vi "Details Display Dialog.vi"(0 "Source":string caption="源", 1 "Start":i32[](array[numeric]) caption="开始", 2 "Length":i32[](array[numeric]) caption="长度", 3 "code":i32 caption="代码", 4 "Show Link":bool caption="显示链接", 5 "Details":string="问题原因" caption="详细信息", 7 "dialog type":T3 caption="对话框类型", 9 "Error or Warning":bool caption="错误或警告", 11 "contname":string="继续" caption="控件名", 12 "stopname":string="停止" caption="停止名", 13 "okname":string="确定" caption="确定名", 14 "Tag Found?":T1 caption="找到标识符？") -> (15 "stop event propagated":bool caption="停止被传递的事件")   [LabVIEW 2018]
uses:
  DialogTypeEnum.ctl
  ErrWarn.ctl
  TagReturnType.ctl
  eventvkey.ctl
panel:
  in  "Search ni.com":bool caption="搜索ni.com"
  in  "truncated message":string="（已删节的源）" caption="删节后消息"
  in  "truncated & CH message":string="（已删节的源；见即时帮助窗口）" caption="删节与CH消息"
  out "Source of Error":string caption="错误来源"
  out "scrollbar text":string caption="滚动条文本"
  in  "Test for size":string caption="大小测试"
  out "text":string caption="文本"
  out "Error or Warning Glyph":T2=TRUE caption="错误或警告图形标记"
  in  "OK":bool caption="确定"
  in  "Stop":bool caption="停止"
  in  "Continue":bool caption="继续"
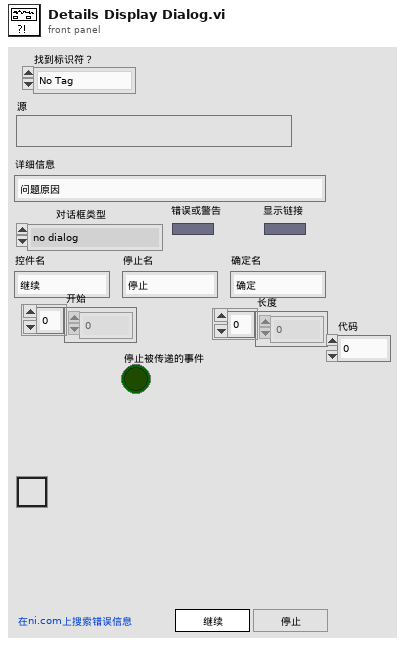
[diagram p1: front panel]
types:
  T1 = typedef "TagReturnType.ctl" = enum16{"No Tag", "<err>", "<append>"}
  T2 = typedef "ErrWarn.ctl" = bool
  T3 = typedef "DialogTypeEnum.ctl" = enum16{"no dialog", "OK message", "continue or stop message", "auto error handling dialog", "OK message + warnings", "continue/stop + warnings"}
  T4 = typedef "eventvkey.ctl" = enum16{"ASCII", "Enter", "Return", "Shift", "Ctrl", "Alt", "Cmd", "Opt", "Caps", "NumLock", "Clear", "Break", "Up", "Down", "Left", "Right", "Insert", "Delete", "Home", "End", "PageUp", "PageDown", "Escape", "Help", "Pause", "ScrollLock", "F1", "F2", "F3", "F4", "F5", "F6", "F7", "F8", "F9", "F10", "F11", "F12", "F13", "F14", "F15", "F16", "F17", "F18", "F19", "F20", "F21", "F22", "F23", "F24", "Play", "VolumeUp", "VolumeDown", "Mute", "Two Byte Char"}
  T5 = typedef "LVRectTypeDef.ctl" = cluster{"Left":i16, "Top":i16, "Right":i16, "Bottom":i16}
  T6 = cluster{"Control":bool, "Shift":bool, "Key":string}
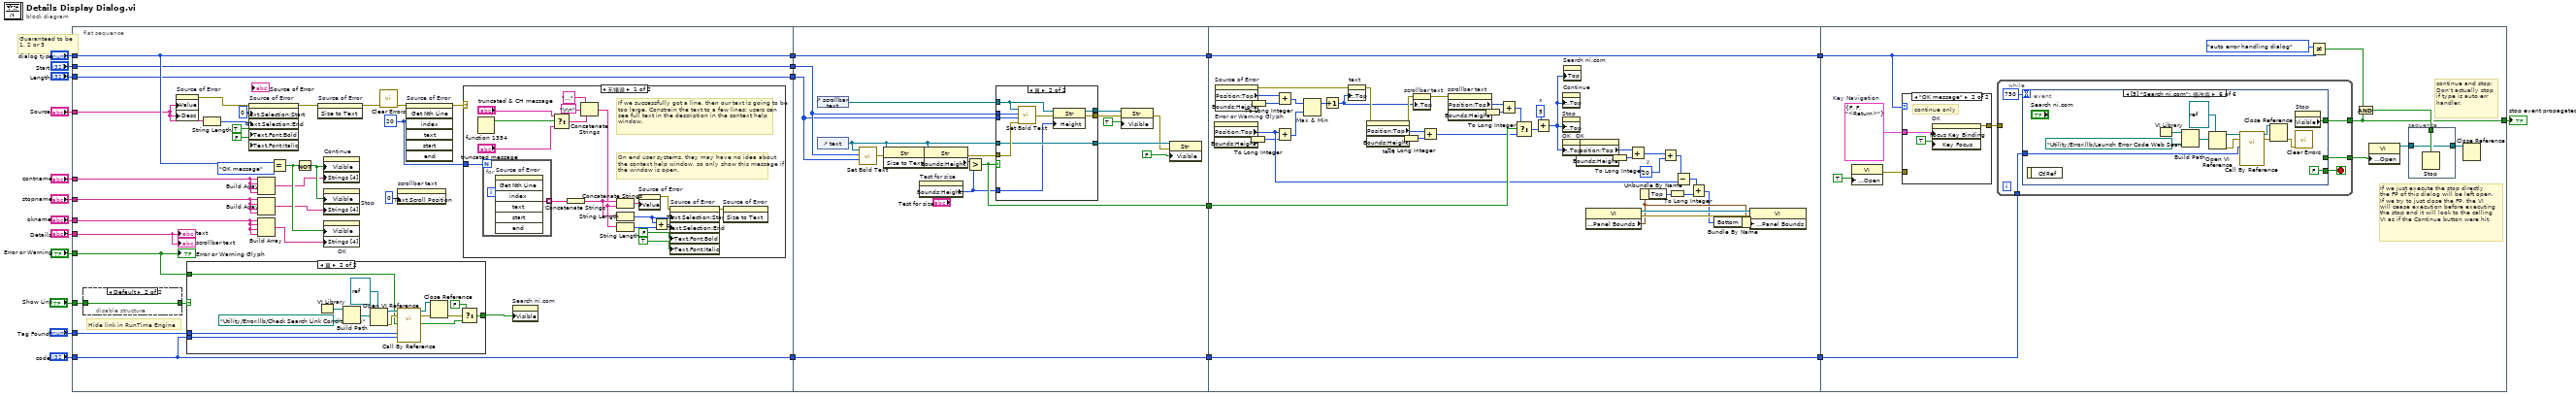
[diagram p0: block diagram]
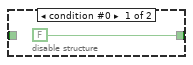
[diagram p2: hidden frame]
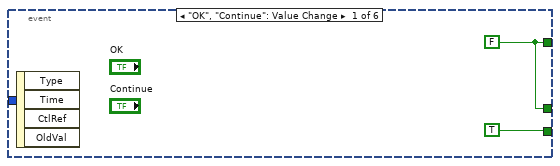
[diagram p6: hidden frame]
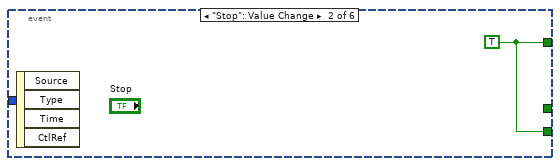
[diagram p7: hidden frame]
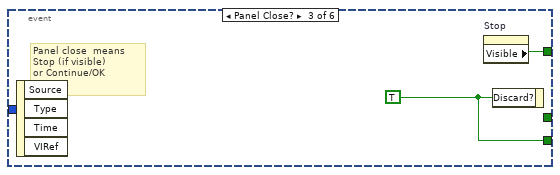
[diagram p8: hidden frame]
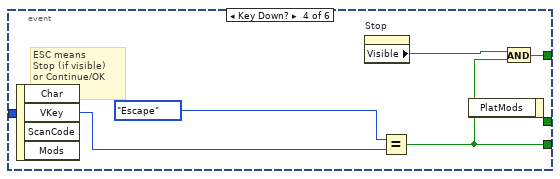
[diagram p9: hidden frame]
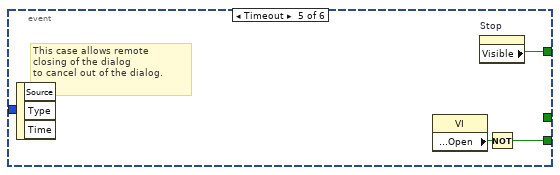
[diagram p10: hidden frame]
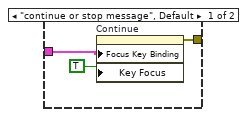
[diagram p11: hidden frame]
diagram:
  # "Guaranteed to be\n1, 2 or 3"
  n1 = flat-sequence {
    tunnel: [w36] -> w21
    tunnel: "dialog type" -> [w36]
    tunnel: "contname" -> [w35]
    tunnel: "stopname" -> [w34]
    tunnel: "okname" -> [w33]
    tunnel: "Source" -> [w29]
    tunnel: "Details" -> [w32]
    tunnel: "Error or Warning" -> [w23]
    tunnel: [w31] -> w10
    tunnel: [w30] -> w9
    tunnel: "Start" -> [w31]
    tunnel: "Length" -> [w30]
    tunnel: "Show Link" -> [w28]
    tunnel: "code" -> [w25]
    tunnel: [w25] -> w2
    tunnel: "Tag Found?" -> [w26]
    tunnel: w21 -> [w94]
    tunnel: [w94] -> w20
    tunnel: [w100] -> w19
    tunnel: w10 -> [w93]
    tunnel: w9 -> [w92]
    tunnel: [w91] -> w3
    tunnel: w2 -> [w91]
    tunnel: w20 -> [w129]
    tunnel: [w129] -> w18
    tunnel: w19 -> [w163]
    tunnel: [w122] -> w4
    tunnel: w3 -> [w122]
    tunnel: [w165] -> w22
    tunnel: w18 -> [w167]
    tunnel: w4 -> [w164]
    frame #0 {
      w43 = u32 20 ("index")
      # "Hide link in RunTime Engine"
      n2 = disable-structure shown="Default" {
        disable-tunnel: w28 -> [_ w55]
        disable-tunnel: [FALSE ("Show Link") w55] -> w27
        frame condition #0 {
        }
        frame condition #1 (active) {
        }
      }
      n3 = property on="Source of Error" class="Str"("Value"=w29, "Desc"=w29) -> (error out=w42:errorcluster)  [unwired: 2 in, 1 out]
      n4 = case shown="真" w27 {
        tunnel: [_ w63] -> w24
        tunnel: w26 -> [_ w62]
        tunnel: w25 -> [_ w61]
        tunnel: w23 -> [_ w60]
        frame False {
        }
        frame True {
          n5 = VI Library() -> (path=w69:path)
          n6 = Build Path(base path=w69, name or relative path=path "Utility/Error.llb/Check Search Link Conditions.vi") -> (appended path=w70:path)
          n7 = Open VI Reference(type specifier VI Refnum (for type only)=refnum<vi> refnum, vi path=w70) -> (vi reference=w66:refnum<vi>, error out=w68:errorcluster)  [unwired: 4 in]
          n8 = call-by-ref "?"(reference=w66, error in=w68, "Error Code"=w61, "Tag Found?"=w62, "Error or Warning?"=w60) -> (reference out=w59:refnum<vi>, error out=w58:errorcluster, "Display Link?"=w65:bool)  [unwired: 8 in]
          n9 = Close Reference(reference=w59, error in (no error)=w58) -> (error out=w57:errorcluster)
          n10 = Select(t=FALSE, s=w57, f=w65) -> (s? t:f=w63:bool)
        }
      }
      n11 = String Length(string=w29) -> (length=w39:i32)
      n12 = property on="Source of Error" class="Str"(error in=w42, "Text.Selection:Start"=u32 0, "Text.Selection:End"=w39, "Text.Font:Bold"=TRUE, "Text.Font:Italic"=FALSE) -> (error out=w41:errorcluster)  [unwired: 1 in, 1 out]
      n13 = Build Array(w35, w35, w35, w35) -> (w51:string[])
      n14 = Build Array(w34, w34, w34, w34) -> (w50:string[])
      n15 = Build Array(w33, w33, w33, w33) -> (w49:string[])
      n16 = Equal?(x=w36, y=DialogTypeEnum."OK message" ("dialog type")) -> (x = y?=w53:bool)
      n17 = Not(x=w53) -> (.not. x?=w52:bool)
      n18 = invoke on="Source of Error" class="Str" method="Size to Text"(error in=w41) -> (error out=w46:errorcluster)  [unwired: 2 in, 2 out]
      n19 = property on="Continue" class="Bool"("Visible"=w52, "Strings [4]"=w51) -> ()  [unwired: 2 in, 2 out]
      n20 = property on="Stop" class="Bool"("Visible"=w52, "Strings [4]"=w50) -> ()  [unwired: 2 in, 2 out]
      n21 = property on="OK" class="Bool"("Visible"=w53, "Strings [4]"=w49) -> ()  [unwired: 2 in, 2 out]
      n22 = call "Clear Errors.vi"("error in (no error)"=w46) -> ("error out"=w45:errorcluster)  [unwired: 5 in, 1 out]
      n23 = property on="scrollbar text" class="Str"("Text.Scroll Position"=u32 0) -> ()  [unwired: 2 in, 2 out]
      n24 = invoke on="Source of Error" class="Str" method="Get Nth Line"(error in=w45, "index"=w43) -> (error out=w44:errorcluster)  [unwired: 5 in, 6 out]
      n25 = case shown="无错误" w44 {
        tunnel: w43 -> [w88 _]
        frame No Error {
          # "If we successfully got a line, then our text is going to be too large. Constrain the text to a few lines; users can see full text in the description in the context help window."
          # "On end user systems, they may have no idea about\nthe context help window, so only show this message if\nthe window is open."
          n26 = fn#1354() -> (1:w78:bool)  [unwired: 1 out]
          n27 = for {
            N: w88 -> [_]
            tunnel: [w89] -> w86 mode=indexing
            i -> [w90]
            n28 = invoke on="Source of Error" class="Str" method="Get Nth Line"("index"=w90) -> ("text"=w89:string)  [unwired: 6 in, 6 out]
          }
          n29 = Select(t="truncated & CH message", s=w78, f="truncated message") -> (s? t:f=w75:string)
          n30 = Concatenate Strings(w86) -> (w85:string)
          n31 = Concatenate Strings("..." ("string"), "\r\n", w75) -> (w72:string)
          n32 = Concatenate Strings(w85, w72) -> (w87:string)
          n33 = String Length(string=w85) -> (length=w80:i32)
          n34 = String Length(string=w72) -> (length=w77:i32)
          n35 = property on="Source of Error" class="Str"("Value"=w87) -> (error out=w82:errorcluster)  [unwired: 2 in, 1 out]
          n36 = Add(x=w80, y=w77) -> (x+y=w79:i32)
          n37 = property on="Source of Error" class="Str"(error in=w82, "Text.Selection:Start"=w80, "Text.Selection:End"=w79, "Text.Font:Bold"=FALSE, "Text.Font:Italic"=TRUE) -> (error out=w81:errorcluster)  [unwired: 1 in, 1 out]
          n38 = invoke on="Source of Error" class="Str" method="Size to Text"(error in=w81) -> ()  [unwired: 2 in, 3 out]
        }
        frame Error {
          # "An error at this point means that there is no line to fetch. That's good. We do not want the text getting too large."
        }
      }
      n39 = property on="Search ni.com" class="Bool"("Visible"=w24) -> ()  [unwired: 2 in, 2 out]
      "Error or Warning Glyph" <- w23
      "scrollbar text" <- w32
      "text" <- w32
    }
    frame #1 {
      n40 = control-ref of="scrollbar text"() -> (w103:refnum<vi>)
      n41 = control-ref of="text"() -> (w95:refnum<vi>)
      n42 = call "Set Bold Text.vi"("Length"=w92, "Start"=w93, "text"=w95) -> ("error out"=w98:errorcluster)  [unwired: 3 in]
      n43 = invoke class="Str" method="Size to Text"(reference=w95, error in=w98) -> (error out=w99:errorcluster)  [unwired: 1 in, 2 out]
      n44 = property on="Test for size" class="Str"() -> ("Bounds:Height"=w97:u32)  [unwired: 2 in, 2 out]
      n45 = property class="Str"(reference=w95, error in=w99) -> (error out=w107:errorcluster, "Bounds:Height"=w108:u32)  [unwired: 1 out]
      n46 = Greater?(x=w108, y=w97) -> (0:w100:bool)
      n47 = case shown="真" w100 {
        tunnel: w107 -> [w111 w120]
        tunnel: w93 -> [_ w119]
        tunnel: w92 -> [_ w118]
        tunnel: [w111 w115] -> w96
        tunnel: w95 -> [w110 w117]
        tunnel: [w110 w112] -> w105
        tunnel: [w109 w117] -> w104
        tunnel: w103 -> [w109 w113]
        tunnel: w97 -> [_ w116]
        frame False {
        }
        frame True {
          n48 = call "Set Bold Text.vi"("error in"=w120, "Length"=w118, "Start"=w119, "text"=w113) -> ("error out"=w114:errorcluster)  [unwired: 2 in]
          n49 = property class="Str"(reference=w113, error in=w114, "Height"=w116) -> (reference out=w112:refnum<vi>, error out=w115:errorcluster)
        }
      }
      n50 = property class="Str"(reference=w105, error in=w96, "Visible"=TRUE ("Defer Panel Updates")) -> (error out=w101:errorcluster)  [unwired: 1 out]
      n51 = property class="Str"(reference=w104, error in=w101, "Visible"=FALSE ("Defer Panel Updates")) -> ()  [unwired: 2 out]
    }
    frame #2 {
      w150 = 20  # y
      w155 = 5  # x
      n52 = property on="Error or Warning Glyph" class="Bool"() -> ("Position:Top"=w145:i32, "Bounds:Height"=w160:u32)  [unwired: 2 in, 2 out]
      n53 = property on="Source of Error" class="Str"() -> (error out=w130:errorcluster, "Position:Top"=w132:i32, "Bounds:Height"=w131:u32)  [unwired: 2 in, 1 out]
      n54 = To Long Integer(number=w160) -> (32bit integer=w128:i32)
      n55 = To Long Integer(number=w131) -> (32bit integer=w127:i32)
      n56 = Add(x=w132, y=w127) -> (x+y=w162:i32)
      n57 = Add(x=w145, y=w128) -> (x+y=w161:i32)
      n58 = Max & Min(x=w162, y=w161) -> (max(x,y)=w159:i32)  [unwired: 1 out]
      n59 = Increment(x=w159) -> (x+1=w138:i32)
      n60 = property on="text" class="Str"(error in=w130, "Position:Top"=w138) -> (error out=w140:errorcluster)  [unwired: 1 in, 1 out]
      n61 = property on="text" class="Str"(error in=w140) -> (error out=w139:errorcluster, "Position:Top"=w137:i32, "Bounds:Height"=w136:u32)  [unwired: 1 in, 1 out]
      n62 = To Long Integer(number=w136) -> (32bit integer=w126:i32)
      n63 = property on="scrollbar text" class="Str"(error in=w139, "Position:Top"=w138) -> (error out=w158:errorcluster)  [unwired: 1 in, 1 out]
      n64 = Add(x=w137, y=w126) -> (x+y=w134:i32)
      n65 = property on="scrollbar text" class="Str"(error in=w158) -> ("Position:Top"=w157:i32, "Bounds:Height"=w156:u32)  [unwired: 1 in, 2 out]
      n66 = To Long Integer(number=w156) -> (32bit integer=w125:i32)
      n67 = Add(x=w157, y=w125) -> (x+y=w135:i32)
      n68 = Select(t=w135, s=w163, f=w134) -> (s? t:f=w133:i32)
      n69 = Add(x=w155, y=w133) -> (x+y=w121:i32)
      n70 = property on="Continue" class="Bool"("Position:Top"=w121) -> ()  [unwired: 2 in, 2 out]
      n71 = property on="Stop" class="Bool"("Position:Top"=w121) -> ()  [unwired: 2 in, 2 out]
      n72 = property on="OK" class="Bool"("Position:Top"=w121) -> (error out=w154:errorcluster)  [unwired: 2 in, 1 out]
      n73 = property on="Search ni.com" class="Bool"("Top"=w121) -> ()  [unwired: 2 in, 2 out]
      n74 = property on="OK" class="Bool"(error in=w154) -> ("Position:Top"=w152:i32, "Bounds:Height"=w153:u32)  [unwired: 1 in, 2 out]
      n75 = property class="VI"() -> (reference out=w147:refnum<vi>, error out=w148:errorcluster, "Front Panel Window:Panel Bounds"=w144:T5)  [unwired: 2 in]
      n76 = To Long Integer(number=w153) -> (32bit integer=w124:i32)
      n77 = Add(x=w152, y=w124) -> (x+y=w151:i32)
      n78 = Unbundle By Name(w144) -> ("Top"=w142:i16)
      n79 = Add(x=w151, y=w150) -> (x+y=w146:i32)
      n80 = To Long Integer(number=w142) -> (32bit integer=w123:i32)
      n81 = Subtract(x=w146, y=w145) -> (x-y=w143:i32)
      n82 = Add(x=w143, y=w123) -> (x+y=w141:i32)
      n83 = Bundle By Name(cluster=w144, "Bottom"=w141) -> (w149:T5)
      n84 = property class="VI"(reference=w147, error in=w148, "Front Panel Window:Panel Bounds"=w149) -> ()  [unwired: 2 out]
    }
    frame #3 {
      w176 = T6 {"Control"=FALSE, "Shift"=FALSE, "Key"="<Return>"}  # Key Navigation
      # "If we just execute the stop directly\nthe FP of this dialog will be left open.\nIf we try to just close the FP, the VI\nwill cease execution before executing\nthe stop and it will look to the calling\nVI as if the Continue button were hit."
      # "continue and stop;\nDon't actually stop\nif type is auto err\nhandler."
      n85 = property class="VI"("Front Panel Window:Open"=TRUE) -> (error out=w175:errorcluster)  [unwired: 2 in, 1 out]
      n86 = case shown="\"OK message\"" w167 {
        tunnel: w176 -> [w211 w214]
        tunnel: w175 -> [_ _]
        tunnel: [w209 w212] -> w173
        frame "continue or stop message", Default {
          n87 = property on="Continue" class="Bool"("Focus Key Binding"=w211, "Key Focus"=TRUE) -> (error out=w209:errorcluster)  [unwired: 2 in, 1 out]
        }
        frame "OK message" {
          # "continue only"
          n88 = property on="OK" class="Bool"("Focus Key Binding"=w214, "Key Focus"=TRUE) -> (error out=w212:errorcluster)  [unwired: 2 in, 1 out]
        }
      }
      n89 = while {
        tunnel: w173 -> [_]
        tunnel: [w182] -> w165
        tunnel: [w181] -> w166
        tunnel: w164 -> [w179]
        stop <- w183 stop-if-true
        n90 = event shown="[5] \"Search ni.com\": 值改变" {
          selector: _ -> [_ _ _ _ _ _]
          dyn-events: _ -> [_ _ _ _ _ _]
          timeout: 750 -> [_ _ _ _ _ _]
          tunnel: [TRUE ("Stop") w186 w188 w189 w194 FALSE ("Discard?")] -> w183
          tunnel: [w185 w186 w187 w192 w196 w208] -> w182
          tunnel: [w185 _ _ _ _ _] -> w181
          tunnel: w179 -> [_ _ _ _ _ w201]
          event "OK", "Continue": Value Change {
            w185 = FALSE ("Stop")
            n91 = event-data() -> ()  [unwired: 1 in, 4 out]
          }
          event "Stop": Value Change {
            w186 = TRUE
            n92 = event-data() -> ()  [unwired: 1 in, 4 out]
          }
          event Panel Close? {
            w188 = TRUE ("Discard?")
            # "Panel close  means\nStop (if visible)\nor Continue/OK"
            n93 = event-data() -> ()  [unwired: 1 in, 4 out]
            n94 = property on="Stop" class="Bool"() -> ("Visible"=w187:bool)  [unwired: 2 in, 2 out]
            n95 = event-data("Discard?"=w188) -> ()  [unwired: 1 in, 1 out]
          }
          event Key Down? {
            # "ESC means\nStop (if visible)\nor Continue/OK"
            n96 = event-data() -> ("VKey"=w191:T4)  [unwired: 1 in, 3 out]
            n97 = property on="Stop" class="Bool"() -> ("Visible"=w193:bool)  [unwired: 2 in, 2 out]
            n98 = Equal?(x=eventvkey."Escape", y=w191) -> (x = y?=w189:bool)
            n99 = event-data() -> ()  [unwired: 2 in, 1 out]
            n100 = And(x=w193, y=w189) -> (x .and. y?=w192:bool)
          }
          event Timeout {
            # "This case allows remote\nclosing of the dialog\nto cancel out of the dialog."
            n101 = event-data() -> ()  [unwired: 1 in, 3 out]
            n102 = property class="VI"() -> ("Front Panel Window:Open"=w195:bool)  [unwired: 2 in, 2 out]
            n103 = property on="Stop" class="Bool"() -> ("Visible"=w196:bool)  [unwired: 2 in, 2 out]
            n104 = Not(x=w195) -> (.not. x?=w194:bool)
          }
          event "Search ni.com": Value Change {
            n105 = event-data() -> ()  [unwired: 1 in, 1 out]
            n106 = VI Library() -> (path=w203:path)
            n107 = Build Path(base path=w203, name or relative path=path "Utility/Error.llb/Launch Error Code Web Search.vi") -> (appended path=w202:path)
            n108 = Open VI Reference(type specifier VI Refnum (for type only)=refnum<vi> refnum, vi path=w202) -> (vi reference=w206:refnum<vi>, error out=w204:errorcluster)  [unwired: 4 in]
            n109 = call-by-ref "?"(reference=w206, error in=w204, "Code"=w201) -> (reference out=w200:refnum<vi>, error out=w199:errorcluster)  [unwired: 11 in]
            n110 = Close Reference(reference=w200, error in (no error)=w199) -> (error out=w198:errorcluster)
            n111 = property on="Stop" class="Bool"() -> ("Visible"=w208:bool)  [unwired: 2 in, 2 out]
            n112 = call "Clear Errors.vi"("error in (no error)"=w198) -> ()  [unwired: 5 in, 2 out]
          }
        }
      }
      n113 = Not Equal?(x=DialogTypeEnum."auto error handling dialog" ("dialog type"), y=w167) -> (x != y?=w172:bool)
      n114 = And(x=w172, y=w165) -> (x .and. y?=w171:bool)
      n115 = property class="VI"("Front Panel Window:Open"=w166) -> (reference out=w169:refnum<vi>)  [unwired: 2 in, 1 out]
      n116 = stacked-sequence {
        tunnel: w169 -> [w177]
        tunnel: w171 -> [w178]
        tunnel: [w177] -> w170
        frame #0 {
          n117 = Stop(stop? (T)=w178) -> ()
        }
      }
      n118 = Close Reference(reference=w170) -> ()  [unwired: 1 in, 1 out]
    }
  }
  "stop event propagated" <- w22
